vi "NavDriveStraight2.vi"(7 "Re-Init":bool, 9 "arguments":string[](array[string]), 10 "SensorInputData":T5, 11 "HMI to Control":T1) -> (2 "HMI to Control Out":T1, 3 "SensorInputDataOut":T5, 4 "Done":bool)   [LabVIEW 2014]
uses:
  Typedefs/SensorInputData.ctl
  Typedefs/HMI_to_Control.ctl
  Typedefs/Arm States.ctl
  Typedefs/ClawStates.ctl
  Typedefs/IntakeWheelSenseOrManual.ctl
panel:
  in  "Yaw_kP":dbl format="%#_13g"
  in  "kP":dbl=1.0 format="%#_13g"
  in  "kI":dbl
  in  "IntegralCap":dbl=0.1 format="%#_13g"
  in  "kD":dbl
  in  "Drive Straight Permissable Error Range":dbl=0.2
  in  "InRangeTimer":i32=200
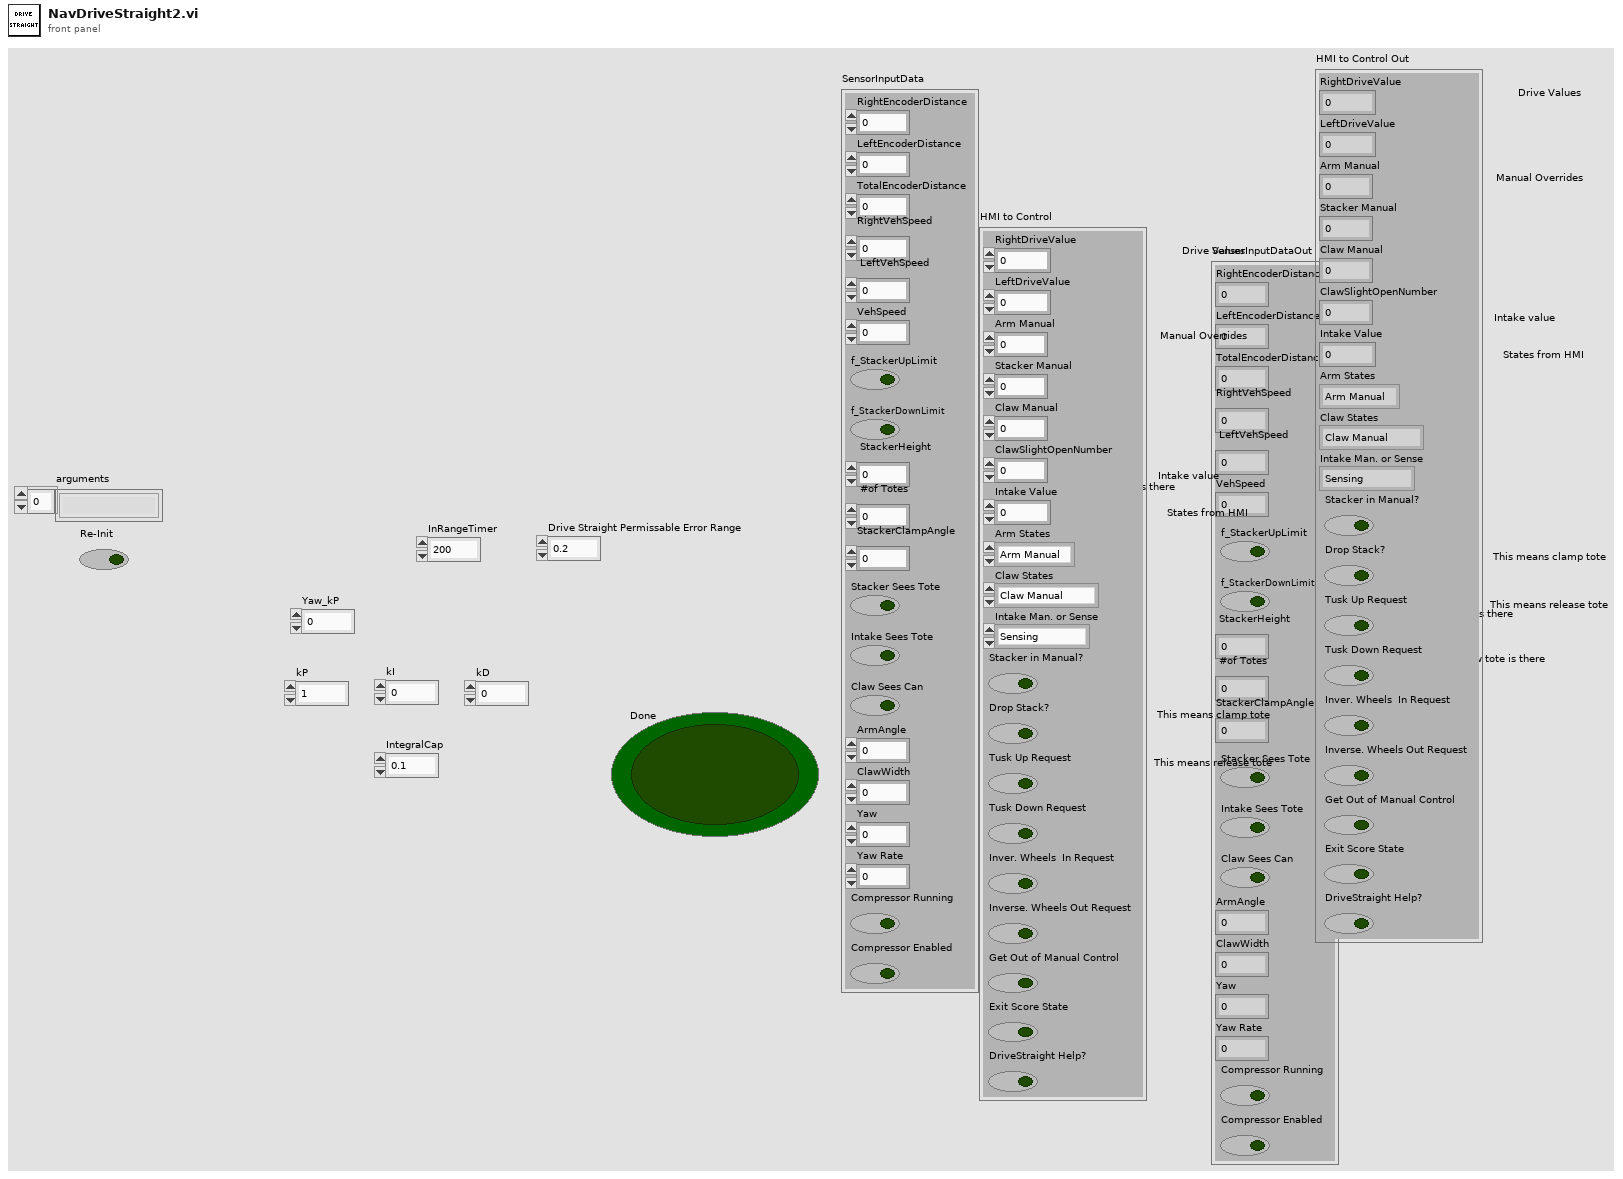
[diagram p1: front panel]
types:
  T1 = typedef "HMI_to_Control.ctl" = cluster{"RightDriveValue":dbl, "LeftDriveValue":dbl, "Arm Manual ":dbl, "Stacker Manual ":dbl, "Claw Manual ":dbl, "ClawSlightOpenNumber":i8, "Intake Value ":i8, "Arm States":T2, "Claw States":T3, "Intake Man. or Sense":T4, "Stacker in Manual?":bool, "Drop Stack? ":bool, "Tusk Up Request":bool, "Tusk Down Request":bool, "Inver. Wheels  In Request":bool, "Inverse. Wheels Out Request ":bool, "Get Out of Manual Control":bool, "Exit Score State":bool, "DriveStraight Help?":bool}
  T2 = typedef "Arm States.ctl" = enum16{"Arm Manual ", "Ground", "Step", "1 Tote", "2 Tote", "3 Tote", "4 Tote", "5 Tote", "6 Tote"}
  T3 = typedef "ClawStates.ctl" = enum16{"Claw Manual ", "Claw Open", "Claw Closed", "Claw Slight Open", "Tote Get"}
  T4 = typedef "IntakeWheelSenseOrManual.ctl" = enum16{"Sensing", "Manual "}
  T5 = typedef "SensorInputData.ctl" = cluster{"RightEncoderDistance":dbl, "LeftEncoderDistance":dbl, "TotalEncoderDistance":dbl, "RightVehSpeed":dbl, "LeftVehSpeed":dbl, "VehSpeed":dbl, "f_StackerUpLimit":bool, "f_StackerDownLimit":bool, "StackerHeight":dbl, "#of Totes":u8, "StackerClampAngle":dbl, "Stacker Sees Tote":bool, "Intake Sees Tote":bool, "Claw Sees Can":bool, "ArmAngle":dbl, "ClawWidth":dbl, "Yaw":dbl, "Yaw Rate":dbl, "Compressor Running":bool, "Compressor Enabled":bool}
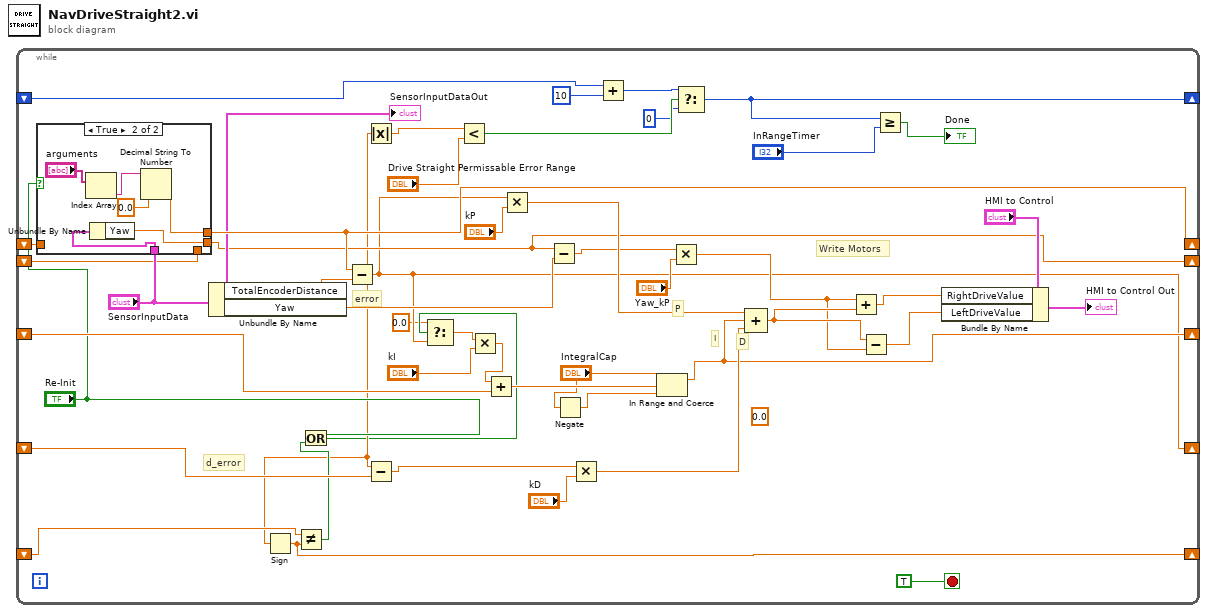
[diagram p0: block diagram]
diagram:
  n1 = while {
    shift-right: [w5] -> _
    shift-left: _ -> [w35]
    shift-right: [w4] -> _
    shift-left: _ -> [w39]
    shift-right: [w27] -> _
    shift-left: _ -> [w29]
    shift-right: [w20] -> _
    shift-left: _ -> [w21]
    shift-right: [w17] -> _
    shift-left: _ -> [w16]
    shift-right: [w13] -> _
    shift-left: _ -> [w12]
    stop <- TRUE stop-if-true
    (unwired) 0.0 ("t")
    # "Write Motors"
    # "D"
    # "d_error"
    # "error"
    # "I"
    # "P"
    n2 = case shown="True" "Re-Init" {
      tunnel: [w49 w52] -> w17
      tunnel: w16 -> [w49 _]
      tunnel: "SensorInputData" -> [_ w51]
      tunnel: [w48 w50] -> w13
      tunnel: w12 -> [w48 _]
      frame False {
      }
      frame True {
        n3 = Index Array(array="arguments") -> (element=w54:string)  [unwired: 1 in]
        n4 = Unbundle By Name(w51) -> ("Yaw"=w50:dbl)
        n5 = Decimal String To Number(string=w54, default (0L)=0.0) -> (number=w52:dbl)  [unwired: 1 in, 1 out]
      }
    }
    n6 = Unbundle By Name("SensorInputData") -> ("TotalEncoderDistance"=w22:dbl, "Yaw"=w15:dbl)
    n7 = Subtract(x=w17, y=w22) -> (x-y=w4:dbl)
    n8 = Sign(1:w4) -> (0:w20:dbl)
    n9 = Not Equal?(x=w21, y=w20) -> (x != y?=w19:bool)
    n10 = Or(x="Re-Init", y=w19) -> (x .or. y?=w2:bool)
    n11 = Absolute Value(x=w4) -> (abs(x)=w34:dbl)
    n12 = Subtract(x=w4, y=w39) -> (x-y=w38:dbl)
    n13 = Select(t=0.0, s=w2, f=w4) -> (s? t:f=w3:dbl)
    n14 = Less?(x=w34, y="Drive Straight Permissable Error Range") -> (x < y?=w32:bool)
    n15 = Multiply(x=w3, y="kI") -> (x*y=w43:dbl)
    n16 = Add(x=w43, y=w35) -> (x+y=w42:dbl)
    n17 = Multiply(x=w4, y="kP") -> (x*y=w45:dbl)
    n18 = Subtract(x=w13, y=w15) -> (x-y=w11:dbl)
    n19 = Negate(x="IntegralCap") -> (-x=w41:dbl)
    n20 = Multiply(x=w38, y="kD") -> (x*y=w36:dbl)
    n21 = Add(x=w29, y=i8 10) -> (x+y=w28:i32)
    n22 = In Range and Coerce(upper limit="IntegralCap", x=w42, lower limit=w41) -> (coerced(x)=w5:dbl)  [unwired: 1 out]
    n23 = Multiply(x=w11, y="Yaw_kP") -> (x*y=w7:dbl)
    n24 = Select(t=w28, s=w32, f=0 ("InRangeTimer 2")) -> (s? t:f=w27:i32)
    n25 = Compound Arithmetic op=ADD(w45, w5, w36) -> (w8:dbl)
    n26 = Add(x=w7, y=w8) -> (x+y=w9:dbl)
    n27 = Subtract(x=w8, y=w7) -> (x-y=w6:dbl)
    n28 = Greater Or Equal?(x=w27, y="InRangeTimer") -> (x >= y?=→"Done":bool)
    n29 = Bundle By Name(cluster="HMI to Control", "RightDriveValue"=w9, "LeftDriveValue"=w6) -> (→"HMI to Control Out":T1)
    "SensorInputDataOut" <- "SensorInputData"
  }
